vi "readTCPDataIn v1.vi"(0 "TCP Network Connection in":refnum<k5>, 5 "Size of data":string, 11 "error in (no error)":errorcluster) -> (4 "TCP Network Connection out":refnum<k5>, 6 "Operation":string, 8 "Size+Operation+Data":T1, 10 "Data":string, 15 "error out":errorcluster)   [LabVIEW 2015]
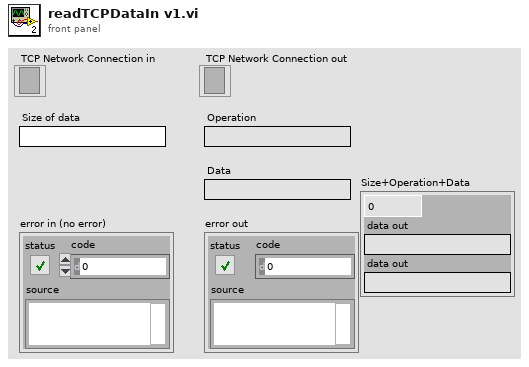
[diagram p1: front panel]
types:
  T1 = cluster{i32, "data out":string, "data out":string}
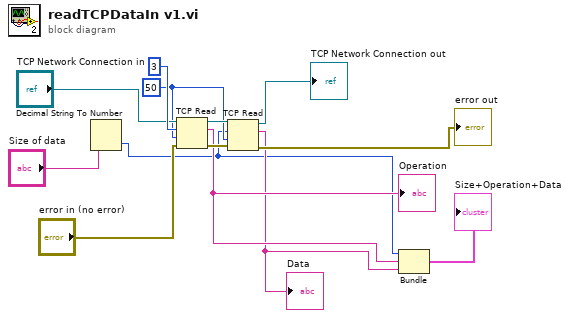
[diagram p0: block diagram]
diagram:
  w6 = 50 ("timeout ms (25000)")
  n1 = Decimal String To Number(string="Size of data") -> (number=w2:i32)  [unwired: 2 in, 1 out]
  n2 = TCP Read(connection ID="TCP Network Connection in", bytes to read=3, error in (no error)="error in (no error)", 9:w6) -> (connection ID out=w9:refnum<k5>, data out=w4:string, error out=w11:errorcluster)  [unwired: 1 in]
  "Operation" <- w4
  n3 = TCP Read(connection ID=w9, bytes to read=w2, error in (no error)=w11, 9:w6) -> (connection ID out=→"TCP Network Connection out":refnum<k5>, data out=w3:string, error out=→"error out":errorcluster)  [unwired: 1 in]
  "Data" <- w3
  n4 = Bundle(w2, "data out"=w4, "data out"=w3) -> (→"Size+Operation+Data":T1)  [unwired: 1 in]
